vi "WriteAttributesTest.vi"() -> ()   [LabVIEW 2014, in "examples.lvlib"]
uses:
  vis/tango_vi.llb/fromStringScalar.vi
  vis/tango_vi.llb/fromShortScalar.vi
  vis/tango_vi.llb/fromLongScalar.vi
  vis/tango_vi.llb/fromDoubleScalar.vi
  examples.lvlib
  vis/tango_vi.llb/tango.lvlib
panel:
  out "success":bool
  in  "value":dbl=23.456
  in  "attribute name":string="double_scalar"
  in  "value":i32=1550
  in  "attribute name":string="long_scalar"
  in  "value":i16=256
  in  "attribute name":string="short_scalar"
  in  "value":string="This is the write value..."
  in  "attribute name":string="string_scalar"
  in  "device name":string="sys/tg_test/1"
  # "TANGO  Binding for LabVIEW - Write Attributes Example"
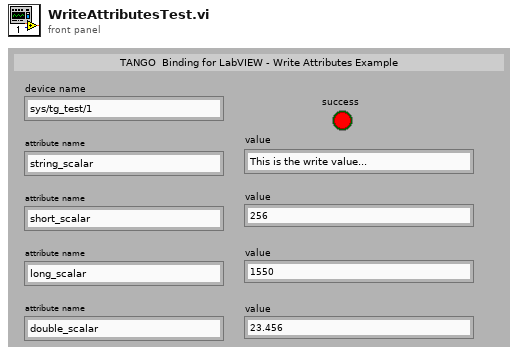
[diagram p1: front panel]
types:
  T1 = typedef "tango.lvlib/_AttributeValue_t.ctl" = cluster{"device name":string, "attribute name":string, "quality value":T2, "quality string":string, "timestamp":dbl, "dim. x":i32, "dim. y":i32, "value":u8[], "error code":i32, "error stack":string[], "data type":T3}
  T2 = typedef "tango.lvlib/_AttributeQuality_t.ctl" = enum16{"VALID", "INVALID", "ALARM", "CHANGING", "UNKNOWN_QUALITY"}
  T3 = typedef "tango.lvlib/_AttributeDataType_t.ctl" = enum16{"STATE_SCA", "STATE_SPE", "STATE_IMG", "STRING_SCA", "STRING_SPE", "STRING_IMG", "BOOL_SCA", "BOOL_SPE", "BOOL_IMG", "UCHAR_SCA", "UCHAR_SPE", "UCHAR_IMG", "SHORT_SCA", "SHORT_SPE", "SHORT_IMG", "USHORT_SCA", "USHORT_SPE", "USHORT_IMG", "LONG_SCA", "LONG_SPE", "LONG_IMG", "ULONG_SCA", "ULONG_SPE", "ULONG_IMG", "LONG64_SCA", "LONG64_SPE", "LONG64_IMG", "ULONG64_SCA", "ULONG64_SPE", "ULONG64_IMG", "FLOAT_SCA", "FLOAT_SPE", "FLOAT_IMG", "DOUBLE_SCA", "DOUBLE_SPE", "DOUBLE_IMG", "ENUM_SCA", "UNKNOWN_DATA_TYPE"}
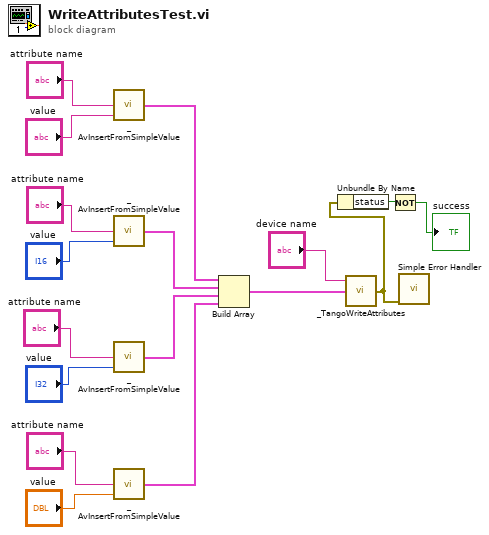
[diagram p0: block diagram]
diagram:
  n1 = call-poly "_AvInsertFromSimpleValue.vi"("value"="value", "attribute name"="attribute name") -> ("attribute value"=w13:T1)  [unwired: 1 in]
  n2 = call-poly "_AvInsertFromSimpleValue.vi"("value"="value", "attribute name"="attribute name") -> ("attribute value"=w11:T1)  [unwired: 1 in]
  n3 = call-poly "_AvInsertFromSimpleValue.vi"("value"="value", "attribute name"="attribute name") -> ("attribute value"=w8:T1)  [unwired: 1 in]
  n4 = call-poly "_AvInsertFromSimpleValue.vi"("value"="value", "attribute name"="attribute name") -> ("attribute value"=w5:T1)  [unwired: 1 in]
  n5 = Build Array(w13, w11, w8, w5) -> (w12:T1[])
  n6 = call "_TangoWriteAttributes.vi"("attribute Values"=w12, "device name"="device name") -> ("error out"=w2:errorcluster)  [unwired: 1 in]
  n7 = Unbundle By Name(w2) -> ("status"=w3:bool)
  n8 = Not(x=w3) -> (.not. x?=→"success":bool)
  n9 = call <vilib>:"Simple Error Handler.vi"("error in (no error)"=w2) -> ()  [unwired: 4 in, 5 out]
